vi "BlinkLED.vi"() -> ()   [LabVIEW 2009]
uses:
  <vilib>/LabVIEW Interface for Arduino/LabVIEW Interface for Arduino.lvlib
  <vilib>/LabVIEW Interface for Arduino/Type Defs/Pin Mode.ctl
panel:
  in  "Stop":bool
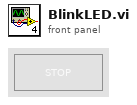
[diagram p1: front panel]
types:
  T1 = typedef "LabVIEW Interface for Arduino.lvlib/Pin Mode.ctl" = enum8{"Input", "Output"}
  T2 = typedef "LabVIEW Interface for Arduino.lvlib/Arduino Resource.ctl" = cluster{"VISA resource":refnum<visa-resource-name>, "Board Type":T3, "Connection Type":enum8{"USB / Serial"}, "Bytes Per Packet (15)":u8}
  T3 = typedef "LabVIEW Interface for Arduino.lvlib/Board Type.ctl" = enum16{"Uno", "Dimuelanove w/Atmega 328", "Mega 2560"}
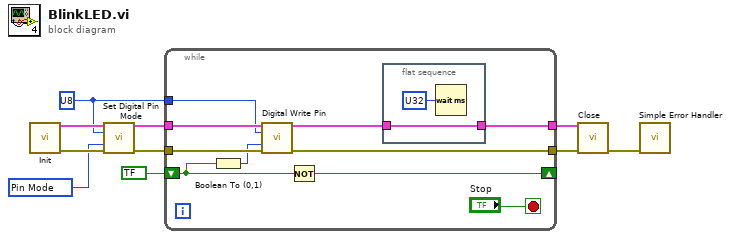
[diagram p0: block diagram]
diagram:
  w1 = u8 ? ("Digital I/O Pin")
  n1 = call <vilib>:"Init.vi"() -> ("Arduino Resource"=w7:T2, "error out"=w6:errorcluster)  [unwired: 18 in]
  n2 = call <vilib>:"Set Digital Pin Mode.vi"("Arduino Resource"=w7, "Digital I/O Pin"=w1, "Pin Mode (Input)"=T1 ?, "error in"=w6) -> ("Arduino Resource"=w5:T2, "error out"=w4:errorcluster)  [unwired: 10 in]
  n3 = while {
    tunnel: [w11] -> w9
    tunnel: w5 -> [w17]
    tunnel: w4 -> [w18]
    tunnel: [w19] -> w8
    tunnel: w1 -> [w16]
    shift-right: [w13] -> _
    shift-left: bool ? -> [w14]
    stop <- "Stop" stop-if-true
    n4 = Boolean To (0,1)(Boolean=w14) -> (0, 1=w15:i16)
    n5 = call <vilib>:"Digital Write Pin.vi"("Arduino Resource"=w17, "Digital I/O Pin (0)"=w16, "Value (0)"=w15, "error in"=w18) -> ("Arduino Resource"=w12:T2, "error out"=w19:errorcluster)  [unwired: 10 in]
    n6 = Not(x=w14) -> (.not. x?=w13:bool)
    n7 = flat-sequence {
      tunnel: w12 -> [w21]
      tunnel: [w21] -> w11
      frame #0 {
        n8 = Wait (ms)(milliseconds to wait=u32 ?) -> ()  [unwired: 1 out]
      }
    }
  }
  n9 = call <vilib>:"Close.vi"("Arduino Resource"=w9, "error in"=w8) -> ("error out"=w10:errorcluster)  [unwired: 13 in]
  n10 = call <vilib>:"Simple Error Handler.vi"("error in (no error)"=w10) -> ()  [unwired: 4 in, 5 out]
